vi "Execute Command.vi"(8 "error in (no error)":errorcluster, 10 "UI Toggle Menu in":refnum<class "UI Toggle Menu.lvclass">, 11 "User Interface References":T1={"This VI"=refnum, "User Interace Plugin"=refnum, "UI Picture Container References"={"Header Image"=refnum, "Footer Image"=refnum}, "Sliding Menu XControl"=refnum, "Menu Container"=refnum, "UI Configuration Information"={"Space Between Buttons"=3, "Number of Buttons to Show"=6, "Header Image"=path "Images/Blue Background.bmp", "Footer Image"=path "Images/Blue Background.bmp"}, "Header Text"=refnum}) -> (0 "error out":errorcluster, 1 "Stop?":bool, 2 "UI Toggle Menu out":refnum<class "UI Toggle Menu.lvclass">, 3 "User Interface References Out":T1={"This VI"=refnum, "User Interace Plugin"=refnum, "UI Picture Container References"={"Header Image"=refnum, "Footer Image"=refnum}, "Sliding Menu XControl"=refnum, "Menu Container"=refnum, "UI Configuration Information"={"Space Between Buttons"=3, "Number of Buttons to Show"=6, "Header Image"=path "Images/Blue Background.bmp", "Footer Image"=path "Images/Blue Background.bmp"}, "Header Text"=refnum})   [LabVIEW 2011, in "UI Toggle Menu.lvclass"]
uses:
  UI Toggle Menu.lvclass
  Main Type Definitions/User Interface Type Definitions.ctl
  Main Type Definitions/UI Picture Containers.ctl
  Sliding Menu/Sliding Menu Library/Sliding Menu xControl/Sliding Menu XControl.xctl
  UI Control Definitions/UI Configuration Information.ctl
  Plugin Handler/Plugin Command Manager/Notify Plugins of Menu Up/Notify Plugins of Menu Up.lvclass
  Plugin Handler/Plugin Command Manager/Notify Plugins of Menu Down/Notify Plugins of Menu Down.lvclass
  Plugin Handler/Plugin Command Manager/Plugin Handler Command.lvclass
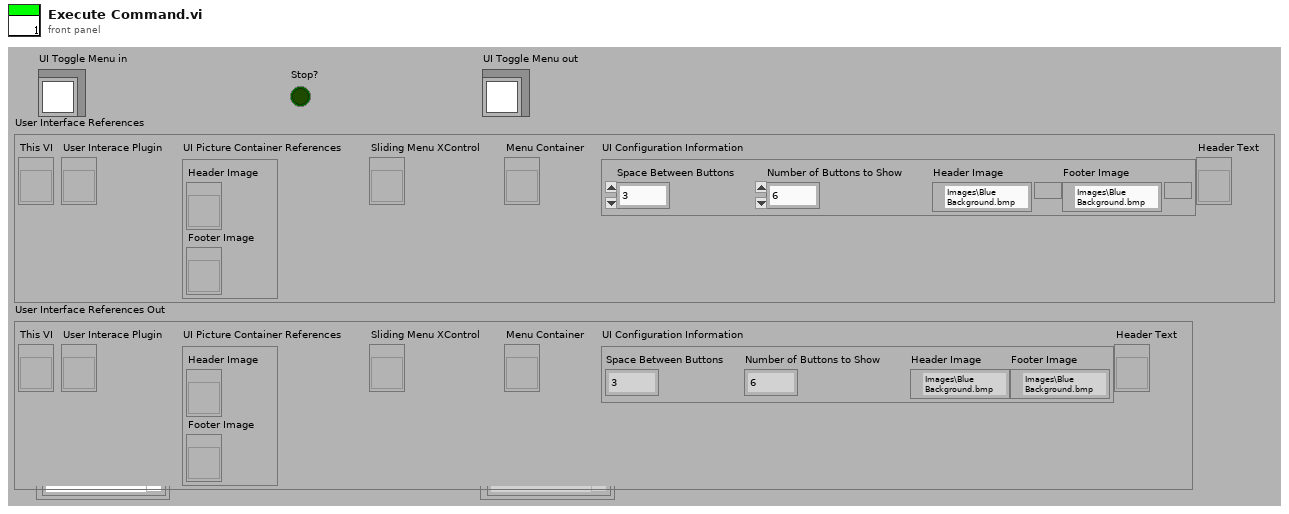
[diagram p1: front panel]
types:
  T1 = typedef "User Interface Type Definitions.ctl" = cluster{"This VI":refnum<vi>, "User Interace Plugin":refnum<vi>, "UI Picture Container References":T2, "Sliding Menu XControl":refnum<vi>, "Menu Container":refnum<vi>, "UI Configuration Information":T3, "Header Text":refnum<vi>}
  T2 = typedef "UI Picture Containers.ctl" = cluster{"Header Image":refnum<vi>, "Footer Image":refnum<vi>}
  T3 = typedef "UI Configuration Information.ctl" = cluster{"Space Between Buttons":i32, "Number of Buttons to Show":i32, "Header Image":path, "Footer Image":path}
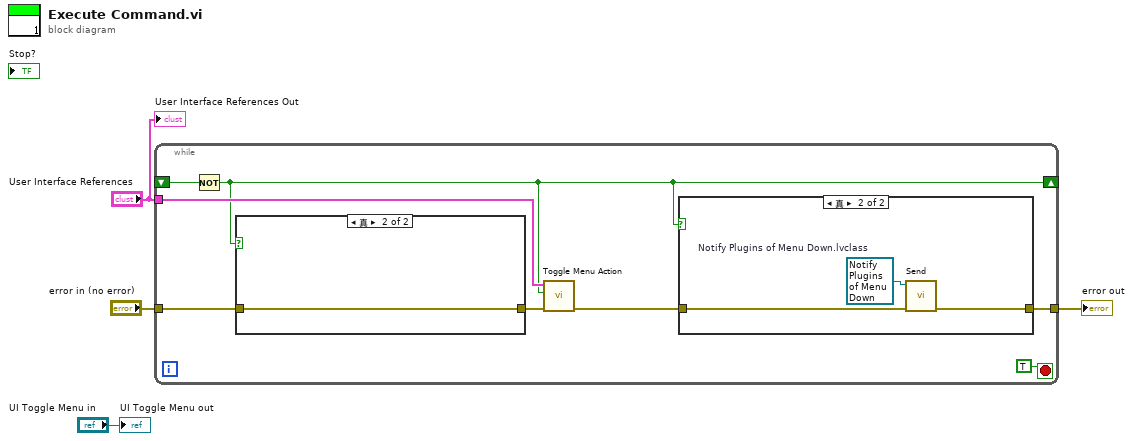
[diagram p0: block diagram]
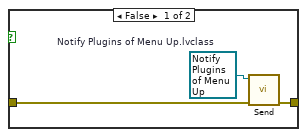
[diagram p2: hidden frame]
diagram:
  n1 = while {
    tunnel: "error in (no error)" -> [w6]
    tunnel: [w8] -> w2
    shift-right: [w7] -> _
    shift-left: _ -> [w10]
    tunnel: "User Interface References" -> [w12]
    stop <- TRUE stop-if-true
    n2 = Not(x=w10) -> (.not. x?=w7:bool)
    n3 = case shown="真" w7 {
      tunnel: w6 -> [w14 w16]
      tunnel: [w13 w16] -> w5
      frame False {
        w15 = refnum<class "Notify Plugins of Menu Up.lvclass"> refnum  # Notify Plugins of Menu Up.lvclass
        n4 = call "Send.vi"("error in (no error)"=w14, "Plugin Generic Command in"=w15) -> ("error out"=w13:errorcluster)  [unwired: 8 in, 1 out]
      }
      frame True {
      }
    }
    n5 = call "Toggle Menu Action.vi"("error in (no error)"=w5, "(T)Down (F) Up"=w7, "User Interface References"=w12) -> ("error out"=w9:errorcluster)  [unwired: 7 in, 1 out]
    n6 = case shown="真" w7 {
      tunnel: w9 -> [w17 w19]
      tunnel: [w17 w18] -> w8
      frame False {
      }
      frame True {
        w20 = refnum<class "Notify Plugins of Menu Down.lvclass"> refnum  # Notify Plugins of Menu Down.lvclass
        n7 = call "Send.vi"("error in (no error)"=w19, "Plugin Generic Command in"=w20) -> ("error out"=w18:errorcluster)  [unwired: 8 in, 1 out]
      }
    }
  }
  "error out" <- w2
  "UI Toggle Menu out" <- "UI Toggle Menu in"
  "User Interface References Out" <- "User Interface References"
